vi "Experimental Triangle Half Ramp.vi"(1 "Phase Offset":dbl format="%#_13g") -> (0 "Half Triangle":waveform(dbl))   [LabVIEW 2013]
uses:
  <vilib>/measure/NI_MABase.lvlib
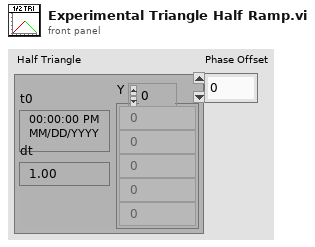
[diagram p1: front panel]
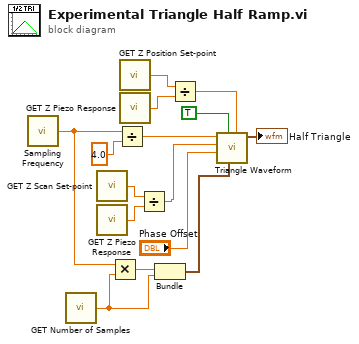
[diagram p0: block diagram]
diagram:
  n1 = call "Sampling Frequency.vi"() -> ("Sampling Frequency"=w2:dbl)
  n2 = call "GET Number of Samples.vi"() -> ("Number of Samples"=w7:dbl)
  n3 = call "GET Z Scan Set-point.vi"() -> ("Z Scan Set-point"=w11:dbl)
  n4 = call "GET Z Piezo Response.vi"() -> ("Z Piezo Response"=w10:dbl)
  n5 = Multiply(x=w2, y=w7) -> (x*y=w6:dbl)
  n6 = Divide(x=w2, y=4.0) -> (x/y=w3:dbl)
  n7 = call "GET Z Position Set-point.vi"() -> ("Z Position Set-point"=w13:dbl)
  n8 = call "GET Z Piezo Response.vi"() -> ("Z Piezo Response"=w14:dbl)
  n9 = Divide(x=w11, y=w10) -> (x/y=w9:dbl)
  n10 = Bundle(w6, "Number of Samples"=w7) -> (w8:cluster{dbl, "Number of Samples":dbl})  [unwired: 1 in]
  n11 = Divide(x=w13, y=w14) -> (x/y=w12:dbl)
  n12 = call <vilib>:"Triangle Waveform.vi"("offset"=w12, "sampling info"=w8, "reset signal"=TRUE, "phase"="Phase Offset", "amplitude"=w9, "frequency"=w3) -> ("signal out"=→"Half Triangle":waveform(dbl))  [unwired: 4 in, 1 out]
